vi "I2C_Open.vi"(5 "Bus":i32=1, 8 "error in":errorcluster) -> (0 "error out":errorcluster)   [LabVIEW 2014]
doc: "Open the specified I2C bus"
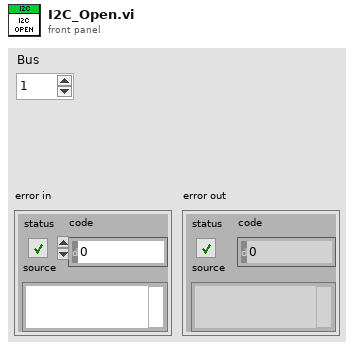
[diagram p1: front panel]
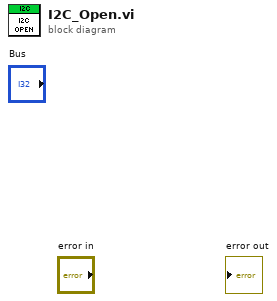
[diagram p0: block diagram]
diagram:
